vi "myRIO_BRig_RT_dataMTrig_Solenoid_c__R.vi"() -> (2 "output_Solenoid_c__R":i32)   [LabVIEW 2014]
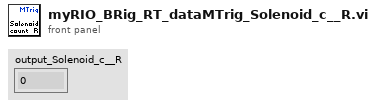
[diagram p1: front panel]
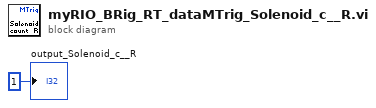
[diagram p0: block diagram]
diagram:
  "output_Solenoid_c__R" <- 1 ("output_iBlock")
